vi "DAC正弦信号生成实验.vi"() -> ()   [LabVIEW 2011]
uses:
  <vilib>/STM32_DriverVI_Interface/DAC/DAC_Buffer_Enable_Interface.ctl
  <vilib>/eio/EIO_TerminalDirection.ctl
  <vilib>/STM32_DriverVI_Interface_F4/DAC/DAC_Channel_Interface_F4.ctl
  <vilib>/STM32_DriverVI_Interface_F4/ADC/ADC123_Period_Interface_F4.ctl
  <vilib>/STM32_DriverVI_Interface/ADC/ADC1_Channel_Interface.ctl
  <vilib>/STM32_DriverVI_Interface_F4/DAC_EIO/DAC_EIO_Interface_F4.vi
  <vilib>/STM32_DriverVI_Interface_F4/ADC_EIO/ADC1_EIO_Interface_F4.vi
  <vilib>/eio/EIONode/EIONode.xnode
panel:
  out "波形图表 2":sgl(graph)
  out "波形图表":dbl(graph)
  in  "F（Hz）":dbl
  in  "停止":bool
  out "度":i32
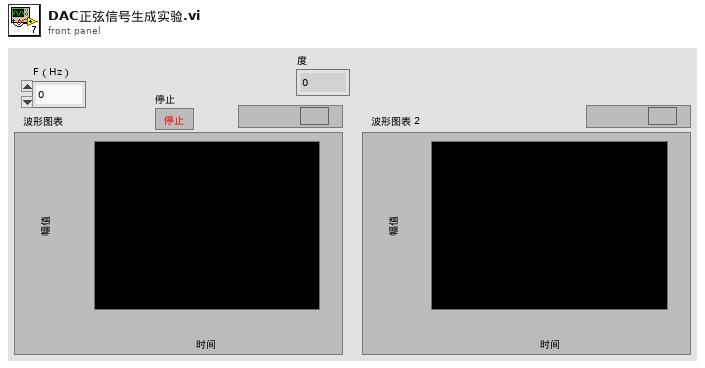
[diagram p1: front panel]
types:
  T1 = typedef "ADC123_Period_Interface_F4.ctl" = enum8{"0.71 us", "1.28 us", "1.90 us", "3.24 us", "4.57 us", "5.90 us", "7.43 us", "23.4 us"}
  T2 = typedef "ADC1_Channel_Interface.ctl" = enum8{"Channel_0（PA0）", "Channel_1（PA1）", "Channel_2（PA2）", "Channel_3（PA3）", "Channel_4（PA4）", "Channel_5（PA5）", "Channel_6（PA6）", "Channel_7（PA7）", "Channel_8（PB0）", "Channel_9（PB1）", "Channel_10（PC0）", "Channel_11（PC1）", "Channel_12（PC2）", "Channel_13（PC3）", "Channel_14（PC4）", "Channel_15（PC5）", "Channel_16（Temperature_Inner）", "Channel_17（Voltage_Ref_Inner）"}
  T3 = typedef "DAC_Buffer_Enable_Interface.ctl" = enum8{"Disable", "Enable"}
  T4 = typedef "DAC_Channel_Interface_F4.ctl" = enum8{"DAC1_Channel（PA4）", "DAC2_Channel（PA5）"}
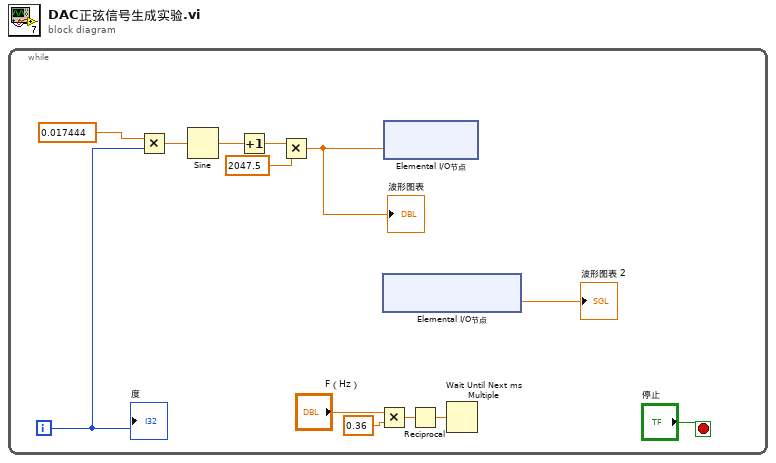
[diagram p0: block diagram]
diagram:
  n1 = while {
    i -> [w11]
    stop <- "停止" stop-if-true
    n2 = Multiply(x=0.017444, y=w11) -> (x*y=w12:dbl)
    n3 = Sine(x=w12) -> (sin(x)=w9:dbl)
    n4 = Increment(x=w9) -> (x+1=w8:dbl)
    n5 = Multiply(x=w8, y=2047.5) -> (x*y=w2:dbl)
    "波形图表" <- w2
    n6 = Multiply(x="F（Hz）", y=0.36) -> (x*y=w4:dbl)
    n7 = xnode "Elemental I/O节点"() -> ("ADC1_Channel_1"=→"波形图表 2":sgl)  [unwired: 1 in, 1 out]
    n8 = xnode "Elemental I/O节点"("DAC_SIN"=w2) -> ()  [unwired: 1 in, 1 out]
    n9 = Reciprocal(x=w4) -> (1/x=w3:dbl)
    n10 = Wait Until Next ms Multiple(millisecond multiple=w3) -> ()  [unwired: 1 out]
    "度" <- w11
  }
